vi "R-W single parameter ini file.vi"(7 "CMD":enum16{"Read", "Write"}(ring), 8 "error in (no error)":errorcluster, 10 "New Value":string, 11 "INI FileFullName":string) -> (0 "error out":errorcluster, 3 "All":string[](array[string]))   [LabVIEW 2021, in "File RW.lvlib"]
doc: "read write single file, single paramter, only for string.\n2019-03-02 22:08:36"
uses:
  File RW.lvlib
  <vilib>/Utility/file.llb/Read Delimited Spreadsheet (string).vi
  <vilib>/Utility/file.llb/Write Delimited Spreadsheet (string).vi
  <userlib>/John_Lib/TopPath/TopPath.lvlib
panel:
  # "产品型号.ini"
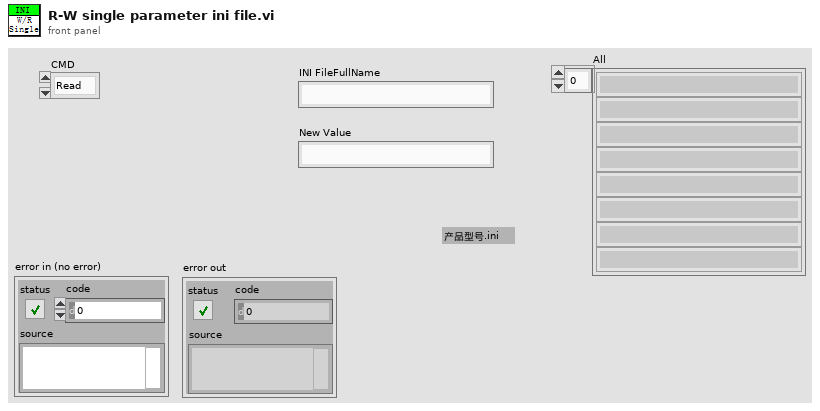
[diagram p1: front panel]
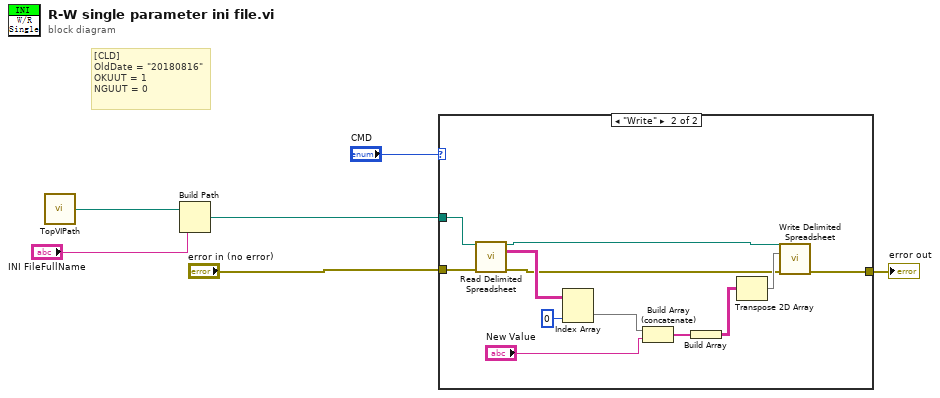
[diagram p0: block diagram]
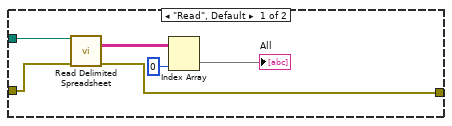
[diagram p2: hidden frame]
diagram:
  # "[CLD]\nOldDate = \"20180816\"\nOKUUT = 1    \nNGUUT = 0"
  n1 = call <userlib>:"TopVIPath.vi"() -> ("ConfigFile path"=w1:path)  [unwired: 2 out]
  n2 = Build Path(base path=w1, name or relative path="INI FileFullName") -> (appended path=w4:path)
  n3 = case shown="\"Write\"" "CMD" {
    tunnel: w4 -> [w12 w17]
    tunnel: "error in (no error)" -> [w8 w19]
    tunnel: [w7 w22] -> w2
    frame "Read", Default {
      n4 = call-poly <vilib>:"Read Delimited Spreadsheet.vi"("file path (dialog if empty)"=w12, "error in (no error)"=w8) -> ("all rows"=w10:string[][], "error out"=w7:errorcluster)  [unwired: 8 in, 4 out]
      n5 = Index Array(array=w10, index (col)=0 ("disabled index (col)")) -> (element=→"All":string[])  [unwired: 1 in]
    }
    frame "Write" {
      n6 = call-poly <vilib>:"Read Delimited Spreadsheet.vi"("file path (dialog if empty)"=w17, "error in (no error)"=w19) -> ("new file path (Not A Path if cancelled)"=w16:path, "all rows"=w20:string[][], "error out"=w18:errorcluster)  [unwired: 8 in, 3 out]
      n7 = Index Array(array=w20, index (col)=0 ("disabled index (col)")) -> (element=w15:string[])  [unwired: 1 in]
      n8 = Build Array (concatenate)(w15, "New Value") -> (w13:string[])
      n9 = Build Array(w13) -> (w23:string[][])
      n10 = Transpose 2D Array(2D array=w23) -> (transposed array=w24:string[][])
      n11 = call-poly <vilib>:"Write Delimited Spreadsheet.vi"("file path (dialog if empty)"=w16, "2D data"=w24, "error in (no error)"=w18) -> ("error out"=w22:errorcluster)  [unwired: 11 in, 1 out]
    }
  }
  "error out" <- w2
